vi "SelectHandle.vi"(8 "error in (no error)":errorcluster, 11 "ClassIn":refnum<class "NiPxi6733.lvclass">) -> (0 "error out":errorcluster, 3 "ClassOut":refnum<class "NiPxi6733.lvclass">)   [LabVIEW 2014, in "FGenPlugins.lvlib" / "NiPxi6733.lvclass"]
uses:
  NiPxi6733.lvclass
  <vilib>/Utility/error.llb/Error Cluster From Error Code.vi
  <vilib>/ErrorRing/Error Ring.xnode
  <resource>/objmgr/daqmx.rc
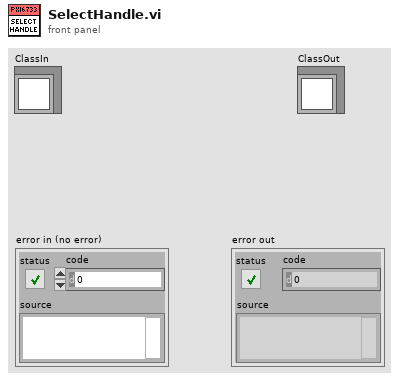
[diagram p1: front panel]
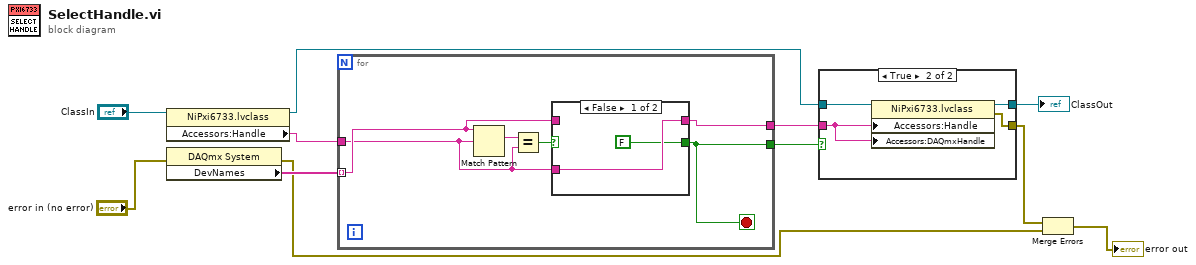
[diagram p0: block diagram]
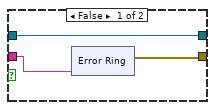
[diagram p2: hidden frame]
diagram:
  n1 = property class="NiPxi6733.lvclass"(reference="ClassIn") -> (reference out=w8:refnum<class "NiPxi6733.lvclass">, "Accessors:Handle"=w9:string)  [unwired: 1 in, 1 out]
  n2 = property class="DAQmx System"(error in="error in (no error)") -> (error out=w1:errorcluster, "DevNames"=w10:tag[])  [unwired: 1 in, 1 out]
  n3 = for {
    tunnel: w10 -> [w15] mode=indexing
    tunnel: w9 -> [w14]
    tunnel: [w13] -> w6
    tunnel: [w12] -> w4
    stop <- w12 stop-if-true
    n4 = Match Pattern(string=w15, regular expression=w14) -> (match substring=w17:string)  [unwired: 1 in, 3 out]
    n5 = Equal?(x=w17, y=w14) -> (x = y?=w16:bool)
    n6 = case shown="False" w16 {
      selector: w16 -> [_ w20]
      tunnel: w15 -> [_ w21]
      tunnel: [w19 w21] -> w13
      tunnel: w14 -> [w19 _]
      tunnel: [FALSE w20] -> w12
      frame False {
      }
      frame True {
      }
    }
  }
  n7 = case shown="True" w4 {
    tunnel: w8 -> [w22 w35]
    tunnel: [w22 w34] -> w7
    tunnel: w6 -> [w23 w33]
    tunnel: [w24 w32] -> w2
    frame False {
      n8 = xnode "Error Ring"("parameter 0"=w23) -> ("error out"=w24:errorcluster)
    }
    frame True {
      n9 = property class="NiPxi6733.lvclass"(reference=w35, "Accessors:Handle"=w33, "Accessors:DAQmxHandle"=w33) -> (reference out=w34:refnum<class "NiPxi6733.lvclass">, error out=w32:errorcluster)  [unwired: 1 in]
    }
  }
  "ClassOut" <- w7
  n10 = Merge Errors(w2, w1) -> (→"error out":errorcluster)
